vi "日志信息出发送队列 (子VI).vi"() -> (0 "错误输出":errorcluster)   [LabVIEW 2016, in "数据传输系统.lvlib"]
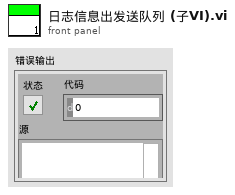
[diagram p1: front panel]
types:
  T1 = enum16{"空白测试", "跨度核查", "标样核查", "加标回收", "平行样", "集成干预"}
  T2 = cluster{"氨氮零点核查索引起始时间":string, "总磷零点核查索引起始时间":string, "总氮零点核查索引起始时间":string, "CODMn零点核查索引起始时间":string, "CODCr零点核查索引起始时间":string, "亚硝酸盐零点核查索引起始时间":string, "硫化物零点核查索引起始时间":string, "ORP零点核查索引起始时间":string}
  T3 = cluster{"数组[0]":string, "数组[1]":string, "数组[2]":string, "数组[3]":string, "数组[4]":string, "数组[5]":string, "数组[6]":string, "数组[7]":string}
  T4 = cluster{"PH":string[][], "CODCr":string[][], "氨氮":string[][], "CODMn":string[][], "总氮":string[][], "总磷":string[][], "电导率":string[][], "水温":string[][], "DO":string[][], "浊度":string[][], "叶绿素":string[][], "藻密度":string[][], "铜":string[][], "盐度":string[][], "水位":string[][], "流速":string[][], "瞬时流量":string[][], "累积流量":string[][], "亚硝酸盐":string[][], "硫化物":string[][], "ORP":string[][], "铅":string[][], "镉":string[][], "锌":string[][], "镍":string[][], "锰":string[][], "汞":string[][], "气温":string[][], "气压":string[][], "风速":string[][], "风向":string[][], "盐度 2":string[][], "磷酸盐":string[][], "硝氮":string[][]}
  T5 = cluster{"氨氮跨度核查索引起始时间":string, "总磷跨度核查索引起始时间":string, "总氮跨度核查索引起始时间":string, "CODMn跨度核查索引起始时间":string, "CODCr跨度核查索引起始时间":string, "亚硝酸盐跨度核查索引起始时间":string, "硫化物跨度核查索引起始时间":string, "ORP跨度核查索引起始时间":string}
  T6 = cluster{"氨氮标样核查索引起始时间":string, "总磷标样核查索引起始时间":string, "总氮标样核查索引起始时间":string, "CODMn标样核查索引起始时间":string, "CODCr标样核查索引起始时间":string, "DO标样核查索引起始时间":string, "PH标样核查索引起始时间":string, "比电导率标样核查索引起始时间":string, "水温标样核查索引起始时间":string, "浊度标样核查索引起始时间":string, "叶绿素a标样核查索引起始时间":string, "藻密度标样核查索引起始时间":string, "亚硝酸盐标样核查索引起始时间":string, "硫化物标样核查索引起始时间":string, "ORP标样核查索引起始时间":string}
  T7 = cluster{"数组[0]":string, "数组[1]":string, "数组[2]":string, "数组[3]":string, "数组[4]":string, "数组[5]":string, "数组[6]":string, "数组[7]":string, "数组[8]":string, "数组[9]":string, "数组[10]":string, "数组[11]":string, "数组[12]":string, "数组[13]":string, "数组[14]":string}
  T8 = cluster{"氨氮加标回收索引起始时间":string, "总磷加标回收索引起始时间":string, "总氮加标回收索引起始时间":string, "CODMn加标回收索引起始时间":string, "CODCr加标回收索引起始时间":string}
  T9 = cluster{"[0]":string, "[1]":string, "[2]":string, "[3]":string, "[4]":string}
  T10 = cluster{"氨氮平行样索引起始时间":string, "总磷平行样索引起始时间":string, "总氮平行样索引起始时间":string, "CODMn平行样索引起始时间":string, "CODCr平行样索引起始时间":string}
  T11 = cluster{"氨氮集成干预索引起始时间":string, "总磷集成干预索引起始时间":string, "总氮集成干预索引起始时间":string, "CODMn集成干预索引起始时间":string, "CODCr集成干预索引起始时间":string, "DO集成干预索引起始时间":string, "PH集成干预索引起始时间":string, "比电导率集成干预索引起始时间":string, "水温集成干预索引起始时间":string, "浊度集成干预索引起始时间":string, "叶绿素a集成干预索引起始时间":string, "藻密度集成干预索引起始时间":string, "亚硝酸盐集成干预索引起始时间":string, "硫化物集成干预索引起始时间":string, "ORP集成干预索引起始时间":string}
  T12 = cluster{"[0]":string, "[1]":string, "[2]":string, "[3]":string, "[4]":string, "[5]":string, "[6]":string, "[7]":string, "[8]":string, "[9]":string, "[10]":string, "[11]":string, "[12]":string, "[13]":string, "[14]":string}
  T13 = cluster{"氨氮仪器日志索引起始时间":string, "总磷仪器日志索引起始时间":string, "总氮仪器日志索引起始时间":string, "CODMn仪器日志索引起始时间":string, "CODCr仪器日志索引起始时间":string, "系统仪器日志索引起始时间":string}
  T14 = cluster{"[0]":string, "[1]":string, "[2]":string, "[3]":string, "[4]":string, "[5]":string}
  T15 = cluster{"氨氮报警信息索引起始时间":string, "总磷报警信息索引起始时间":string, "总氮报警信息索引起始时间":string, "CODMn报警信息索引起始时间":string, "CODCr报警信息索引起始时间":string, "DO报警信息索引起始时间":string, "PH报警信息索引起始时间":string, "比电导率报警信息索引起始时间":string, "水温报警信息索引起始时间":string, "浊度报警信息索引起始时间":string, "叶绿素报警信息索引起始时间":string, "系统报警信息索引起始时间":string}
  T16 = cluster{"[0]":string, "[1]":string, "[2]":string, "[3]":string, "[4]":string, "[5]":string, "[6]":string, "[7]":string, "[8]":string, "[9]":string, "[10]":string, "[11]":string}
  T17 = cluster{"氨氮仪器参数索引起始时间":string, "总磷仪器参数索引起始时间":string, "总氮仪器参数索引起始时间":string, "CODMn仪器参数索引起始时间":string, "CODCr仪器参数索引起始时间":string, "DO仪器参数索引起始时间":string, "PH仪器参数索引起始时间":string, "比电导率仪器参数索引起始时间":string, "水温仪器参数索引起始时间":string, "浊度仪器参数索引起始时间":string, "叶绿素a仪器参数索引起始时间":string, "藻密度仪器参数索引起始时间":string, "ORP仪器参数索引起始时间":string}
  T18 = cluster{"[0]":string, "[1]":string, "[2]":string, "[3]":string, "[4]":string, "[5]":string, "[6]":string, "[7]":string, "[8]":string, "[9]":string, "[10]":string, "[11]":string, "[12]":string}
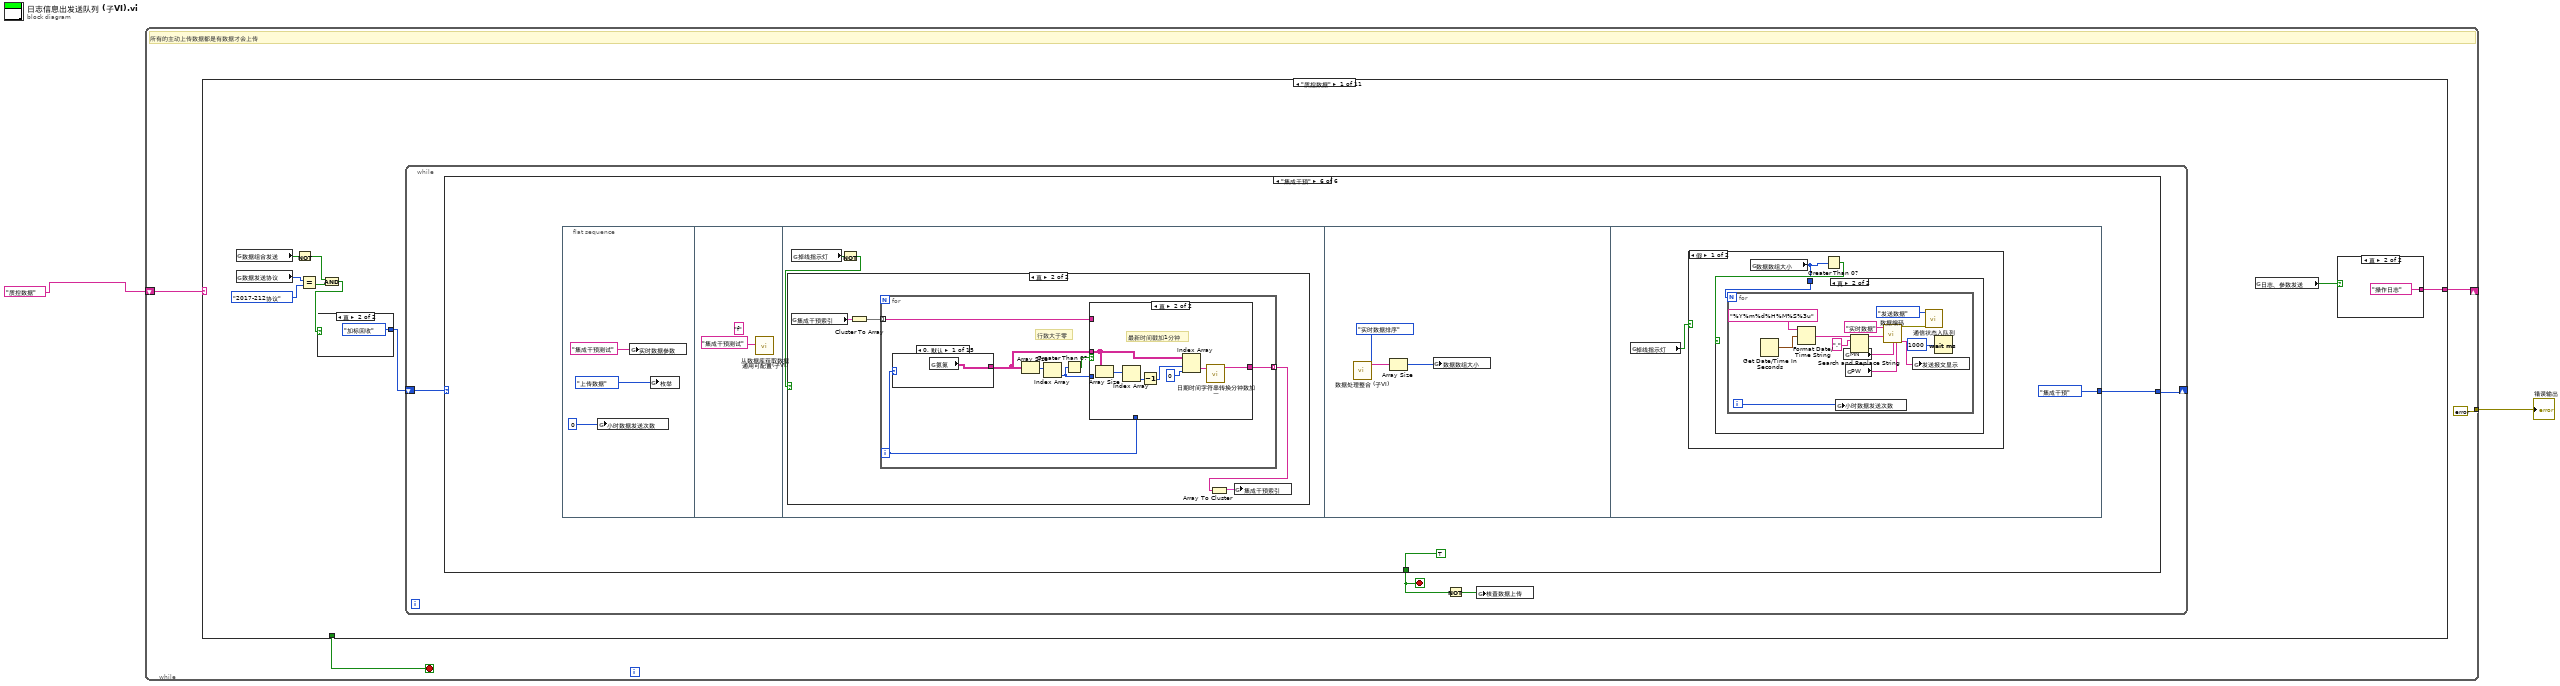
[diagram p0: block diagram]
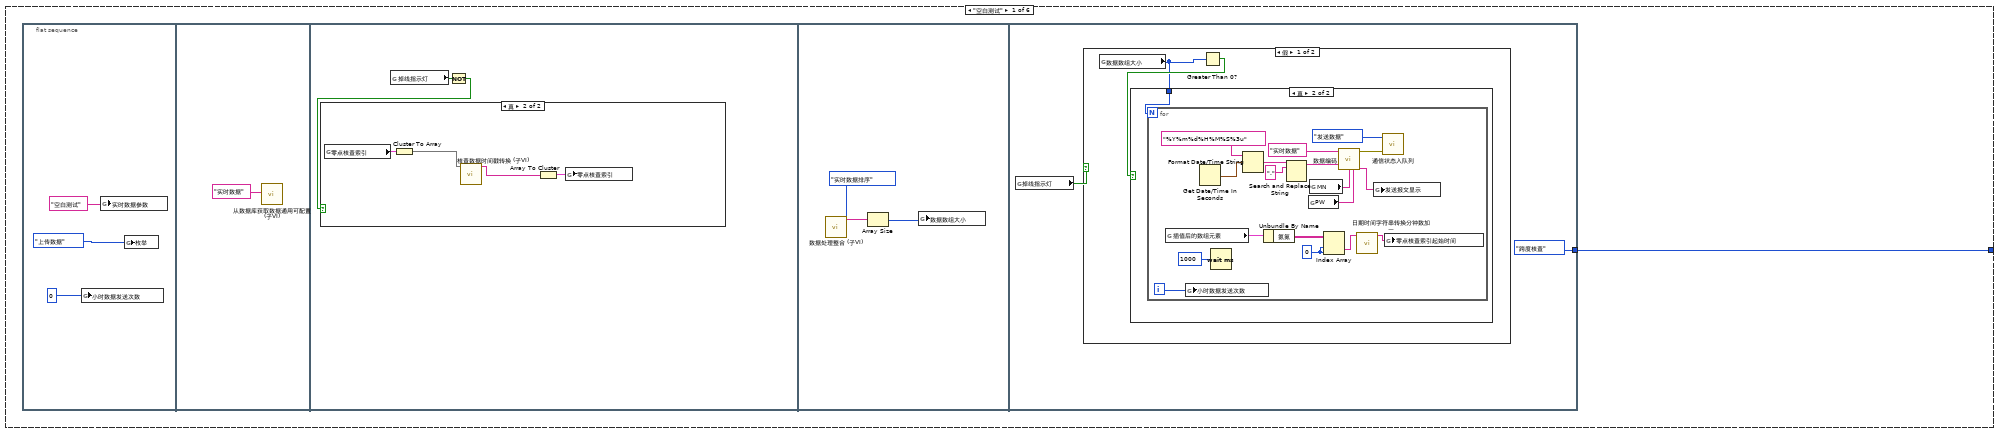
[diagram p2: hidden frame]
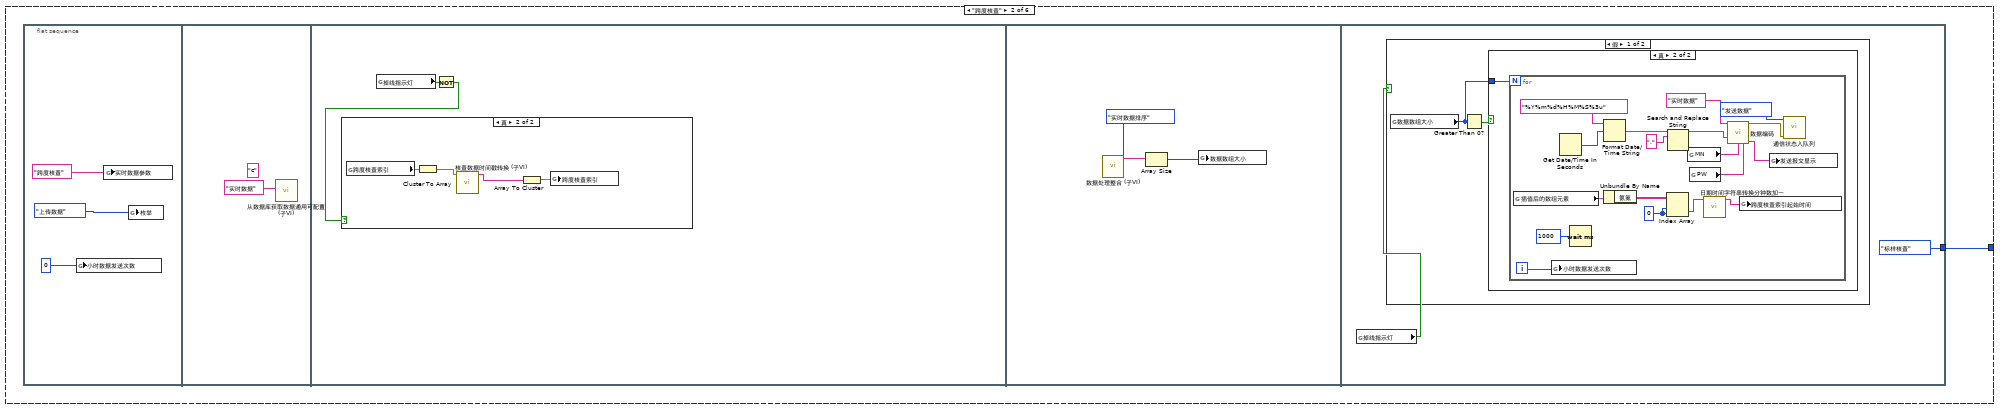
[diagram p6: hidden frame]
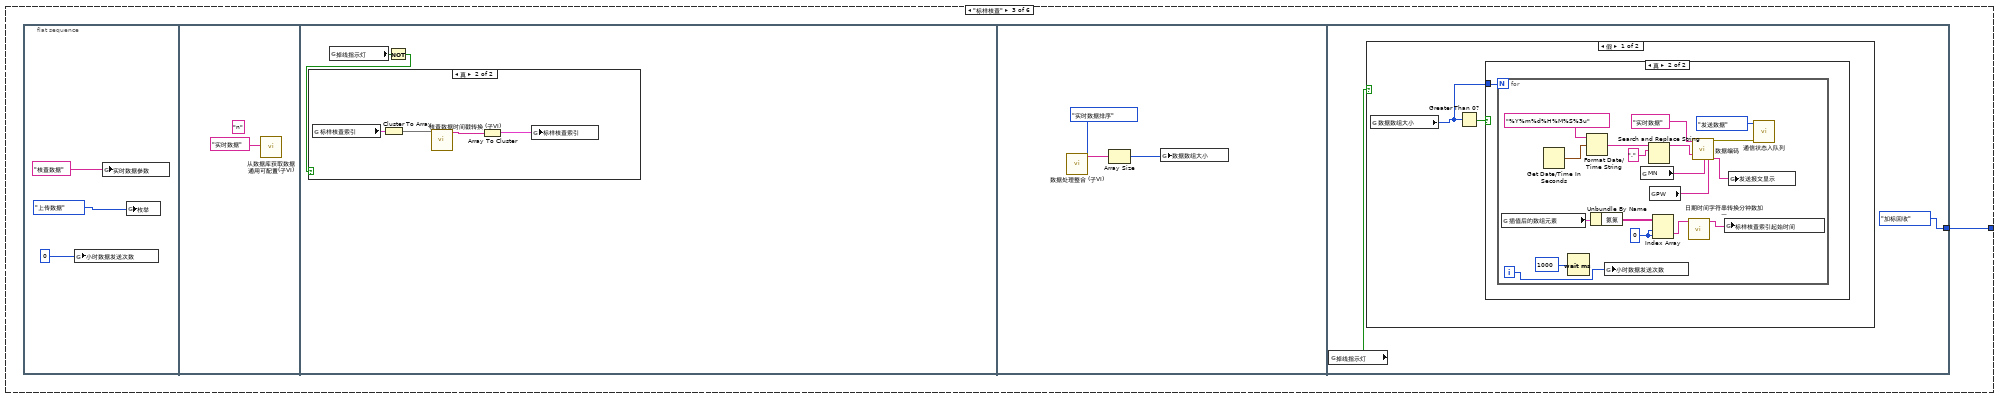
[diagram p10: hidden frame]
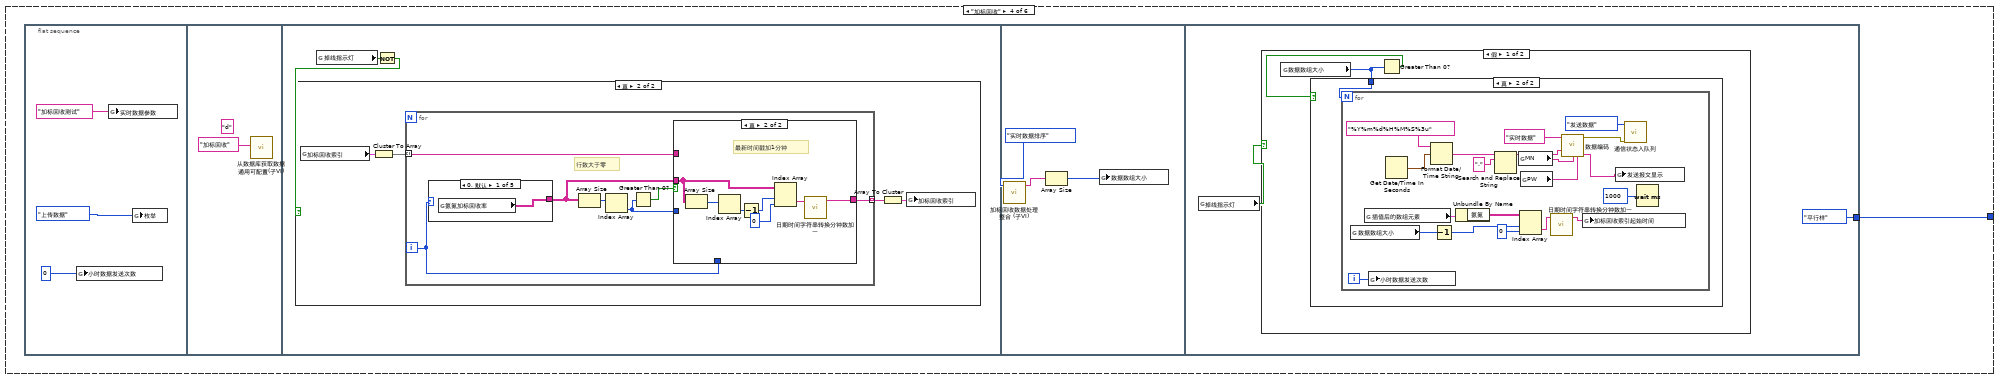
[diagram p14: hidden frame]
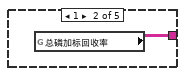
[diagram p16: hidden frame]
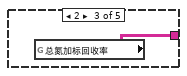
[diagram p17: hidden frame]
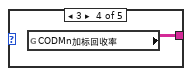
[diagram p18: hidden frame]
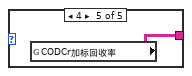
[diagram p19: hidden frame]
diagram:
  n1 = while "While循环" {
    shift-right: [w5] -> _
    shift-left: "质控数据" ("组合框") -> [w6]
    tunnel: [errorcluster {"status"=FALSE, "code"=0, "source"=""} ("错误输出")] -> w2
    stop <- w3 stop-if-true
    # "所有的主动上传数据都是有数据才会上传"
    n2 = case shown="\"质控数据\"" w6 {
      tunnel: [w15 w309 "系统状态" ("组合框") w410 "测量周期" ("组合框") "超标留样" ("组合框") "报警信息" ("组合框") w504 w569 "环境参数" ("组合框") "环境参数" ("组合框")] -> w5
      tunnel: [_ _ _ _ _ _ _ _ _ _ TRUE] -> w3
      frame "质控数据" {
        n3 = global read "断电保存全局.vi" "数据组合发送"() -> (w10:bool)
        n4 = global read "断电保存全局.vi" "数据发送协议"() -> (w13:enum16{"2005-212协议", "2017-212协议"})
        n5 = Not(x=w10) -> (.not. x?=w9:bool)
        n6 = Equal?(x=w13, y=enum16{"2005-212协议", "2017-212协议"}."2017-212协议" ("数据发送协议")) -> (x = y?=w11:bool)
        n7 = And(x=w9, y=w11) -> (x .and. y?=w8:bool)
        n8 = case shown="真" w8 {
          tunnel: [T1."空白测试" T1."加标回收"] -> w7
          frame False {
          }
          frame True {
          }
        }
        n9 = while {
          shift-right: [w18] -> _
          shift-left: w7 -> [w19]
          stop <- w16 stop-if-true
          n10 = case shown="\"集成干预\"" w19 {
            tunnel: [_ _ _ _ _ TRUE] -> w16
            tunnel: [w20 w57 w94 w131 w190 w242] -> w18
            frame "空白测试" {
              n11 = flat-sequence {
                tunnel: [T1."跨度核查"] -> w20
                frame #0 {
                  n12 = global write "全局 小时数据发送次数.vi" "小时数据发送次数"(0 ("小时数据发送次数")) -> ()
                  n13 = global write "全局 实时数据参数.vi" "实时数据参数"("空白测试") -> ()
                  n14 = global write "全局1.vi" "枚举"(enum16{"返回请求应答", "上传数据", "返回执行结果"}."上传数据" ("枚举")) -> ()
                }
                frame #1 {
                  n15 = call "从数据库获取数据通用可配置(子VI).vi"("table输入"="实时数据" ("新元素/子数组")) -> ()  [unwired: 9 in, 2 out]
                }
                frame #2 {
                  n16 = global read "全局 数据发送重叠.vi" "掉线指示灯"() -> (w26:bool)
                  n17 = Not(x=w26) -> (.not. x?=w25:bool)
                  n18 = case shown="真" w25 {
                    frame False {
                    }
                    frame True {
                      n19 = global read "全局 时间2.vi" "零点核查索引"() -> (w30:T2)
                      n20 = Cluster To Array(cluster=w30) -> (array=w28:string[])
                      n21 = call "核查数据时间戳转换 (子VI).vi"("核查索引"=w28) -> ("数组"=w27:string[])  [unwired: 10 in]
                      n22 = Array To Cluster(array=w27) -> (cluster=w29:T3)
                      n23 = global write "全局 时间2.vi" "零点核查索引"(w29) -> ()
                    }
                  }
                }
                frame #3 {
                  n24 = call "数据处理整合 (子VI).vi"("枚举"=enum16{"实时数据排序", "小时数据排序"}."实时数据排序") -> ("已排序的数组"=w33:string[])  [unwired: 10 in]
                  n25 = Array Size(array=w33) -> (size(s)=w32:i32)
                  n26 = global write "全局 数据数组大小.vi" "数据数组大小"(w32) -> ()
                }
                frame #4 {
                  n27 = global read "全局 数据发送重叠.vi" "掉线指示灯"() -> (w35:bool)
                  n28 = case shown="假" w35 {
                    frame False {
                      n29 = global read "全局 数据数组大小.vi" "数据数组大小"() -> (w36:i32)
                      n30 = Greater Than 0?(x=w36) -> (x > 0?=w37:bool)
                      n31 = case shown="真" w37 {
                        tunnel: w36 -> [_ w38]
                        frame False {
                        }
                        frame True {
                          n32 = for {
                            N: w38 -> [_]
                            i -> [w39]
                            w51 = 0 ("禁用的索引 (列)")
                            n33 = global read "插值后的新数组.vi" "插值后的数组元素"() -> (w55:T4)
                            n34 = global write "全局 小时数据发送次数.vi" "小时数据发送次数"(w39) -> ()
                            n35 = Get Date/Time In Seconds() -> (seconds since 1Jan1904=w43:timestamp)
                            n36 = Wait (ms)(milliseconds to wait=u32 1000 ("等待时间（毫秒）")) -> ()  [unwired: 1 out]
                            n37 = Format Date/Time String(time format string (%c)="%Y%m%d%H%M%S%3u" ("时间格式字符串(%c)"), seconds (now)=w43) -> (date/time string=w42:string)  [unwired: 1 in]
                            n38 = Unbundle By Name(w55) -> ("氨氮"=w54:string[][])
                            n39 = Search and Replace String(input string=w42, search string="." ("搜索字符串")) -> (result string=w40:string)  [unwired: 6 in, 3 out]
                            n40 = global read "断电保存全局.vi" "PW"() -> (w47:string)
                            n41 = global read "断电保存全局.vi" "MN"() -> (w48:string)
                            n42 = Index Array(array=w54, index (row)=w51, index (col)=w51) -> (element=w53:string)
                            n43 = call "数据编码.vi"("table输入"="实时数据" ("新元素/子数组"), "QN"=w40, "MN"=w48, "PW"=w47) -> ("错误常量"=w46:errorcluster, "通讯包字符串"=w50:string)  [unwired: 10 in]
                            n44 = call "日期时间字符串转换分钟数加一.vi"("data[0]"=w53) -> ("日期/时间字符串"=w52:string)  [unwired: 10 in]
                            n45 = global write "全局1.vi" "发送报文显示"(w50) -> ()
                            n46 = call "通信状态入队列.vi"("错误输入（无错误）"=w46, "枚举"=enum16{"打开连接", "发送数据", "读取数据", "数据处理", "关闭连接"}."发送数据") -> ()  [unwired: 9 in, 1 out]
                            n47 = global write "全局 时间2.vi" "零点核查索引起始时间"(w52) -> ()
                          }
                        }
                      }
                    }
                    frame True {
                    }
                  }
                }
              }
            }
            frame "跨度核查" {
              n48 = flat-sequence {
                tunnel: [T1."标样核查"] -> w57
                frame #0 {
                  n49 = global write "全局 小时数据发送次数.vi" "小时数据发送次数"(0 ("小时数据发送次数")) -> ()
                  n50 = global write "全局 实时数据参数.vi" "实时数据参数"("跨度核查") -> ()
                  n51 = global write "全局1.vi" "枚举"(enum16{"返回请求应答", "上传数据", "返回执行结果"}."上传数据" ("枚举")) -> ()
                }
                frame #1 {
                  (unwired) "c" ("列队名（唯一）")
                  n52 = call "从数据库获取数据通用可配置(子VI).vi"("table输入"="实时数据" ("新元素/子数组")) -> ()  [unwired: 9 in, 2 out]
                }
                frame #2 {
                  n53 = global read "全局 数据发送重叠.vi" "掉线指示灯"() -> (w63:bool)
                  n54 = Not(x=w63) -> (.not. x?=w62:bool)
                  n55 = case shown="真" w62 {
                    frame False {
                    }
                    frame True {
                      n56 = global read "全局 时间2.vi" "跨度核查索引"() -> (w67:T5)
                      n57 = Cluster To Array(cluster=w67) -> (array=w65:string[])
                      n58 = call "核查数据时间戳转换 (子VI).vi"("核查索引"=w65) -> ("数组"=w64:string[])  [unwired: 10 in]
                      n59 = Array To Cluster(array=w64) -> (cluster=w66:T3)
                      n60 = global write "全局 时间2.vi" "跨度核查索引"(w66) -> ()
                    }
                  }
                }
                frame #3 {
                  n61 = call "数据处理整合 (子VI).vi"("枚举"=enum16{"实时数据排序", "小时数据排序"}."实时数据排序") -> ("已排序的数组"=w70:string[])  [unwired: 10 in]
                  n62 = Array Size(array=w70) -> (size(s)=w69:i32)
                  n63 = global write "全局 数据数组大小.vi" "数据数组大小"(w69) -> ()
                }
                frame #4 {
                  n64 = global read "全局 数据发送重叠.vi" "掉线指示灯"() -> (w72:bool)
                  n65 = case shown="假" w72 {
                    frame False {
                      n66 = global read "全局 数据数组大小.vi" "数据数组大小"() -> (w73:i32)
                      n67 = Greater Than 0?(x=w73) -> (x > 0?=w74:bool)
                      n68 = case shown="真" w74 {
                        tunnel: w73 -> [_ w75]
                        frame False {
                        }
                        frame True {
                          n69 = for {
                            N: w75 -> [_]
                            i -> [w76]
                            w88 = 0 ("禁用的索引 (列)")
                            n70 = global read "插值后的新数组.vi" "插值后的数组元素"() -> (w92:T4)
                            n71 = global write "全局 小时数据发送次数.vi" "小时数据发送次数"(w76) -> ()
                            n72 = Get Date/Time In Seconds() -> (seconds since 1Jan1904=w80:timestamp)
                            n73 = Wait (ms)(milliseconds to wait=u32 1000 ("等待时间（毫秒）")) -> ()  [unwired: 1 out]
                            n74 = Format Date/Time String(time format string (%c)="%Y%m%d%H%M%S%3u" ("时间格式字符串(%c)"), seconds (now)=w80) -> (date/time string=w79:string)  [unwired: 1 in]
                            n75 = Unbundle By Name(w92) -> ("氨氮"=w91:string[][])
                            n76 = Index Array(array=w91, index (row)=w88, index (col)=w88) -> (element=w90:string)
                            n77 = Search and Replace String(input string=w79, search string="." ("搜索字符串")) -> (result string=w77:string)  [unwired: 6 in, 3 out]
                            n78 = global read "断电保存全局.vi" "MN"() -> (w86:string)
                            n79 = global read "断电保存全局.vi" "PW"() -> (w85:string)
                            n80 = call "日期时间字符串转换分钟数加一.vi"("data[0]"=w90) -> ("日期/时间字符串"=w89:string)  [unwired: 10 in]
                            n81 = call "数据编码.vi"("table输入"="实时数据" ("新元素/子数组"), "QN"=w77, "MN"=w86, "PW"=w85) -> ("错误常量"=w83:errorcluster, "通讯包字符串"=w84:string)  [unwired: 10 in]
                            n82 = global write "全局 时间2.vi" "跨度核查索引起始时间"(w89) -> ()
                            n83 = global write "全局1.vi" "发送报文显示"(w84) -> ()
                            n84 = call "通信状态入队列.vi"("错误输入（无错误）"=w83, "枚举"=enum16{"打开连接", "发送数据", "读取数据", "数据处理", "关闭连接"}."发送数据") -> ()  [unwired: 9 in, 1 out]
                          }
                        }
                      }
                    }
                    frame True {
                    }
                  }
                }
              }
            }
            frame "标样核查" {
              n85 = flat-sequence {
                tunnel: [T1."加标回收"] -> w94
                frame #0 {
                  n86 = global write "全局 小时数据发送次数.vi" "小时数据发送次数"(0 ("小时数据发送次数")) -> ()
                  n87 = global write "全局 实时数据参数.vi" "实时数据参数"("核查数据") -> ()
                  n88 = global write "全局1.vi" "枚举"(enum16{"返回请求应答", "上传数据", "返回执行结果"}."上传数据" ("枚举")) -> ()
                }
                frame #1 {
                  (unwired) "n" ("列队名（唯一）")
                  n89 = call "从数据库获取数据通用可配置(子VI).vi"("table输入"="实时数据" ("新元素/子数组")) -> ()  [unwired: 9 in, 2 out]
                }
                frame #2 {
                  n90 = global read "全局 数据发送重叠.vi" "掉线指示灯"() -> (w100:bool)
                  n91 = Not(x=w100) -> (.not. x?=w99:bool)
                  n92 = case shown="真" w99 {
                    frame False {
                    }
                    frame True {
                      n93 = global read "全局 时间2.vi" "标样核查索引"() -> (w104:T6)
                      n94 = Cluster To Array(cluster=w104) -> (array=w102:string[])
                      n95 = call "核查数据时间戳转换 (子VI).vi"("核查索引"=w102) -> ("数组"=w101:string[])  [unwired: 10 in]
                      n96 = Array To Cluster(array=w101) -> (cluster=w103:T7)
                      n97 = global write "全局 时间2.vi" "标样核查索引"(w103) -> ()
                    }
                  }
                }
                frame #3 {
                  n98 = call "数据处理整合 (子VI).vi"("枚举"=enum16{"实时数据排序", "小时数据排序"}."实时数据排序") -> ("已排序的数组"=w107:string[])  [unwired: 10 in]
                  n99 = Array Size(array=w107) -> (size(s)=w106:i32)
                  n100 = global write "全局 数据数组大小.vi" "数据数组大小"(w106) -> ()
                }
                frame #4 {
                  n101 = global read "全局 数据发送重叠.vi" "掉线指示灯"() -> (w109:bool)
                  n102 = case shown="假" w109 {
                    frame False {
                      n103 = global read "全局 数据数组大小.vi" "数据数组大小"() -> (w110:i32)
                      n104 = Greater Than 0?(x=w110) -> (x > 0?=w111:bool)
                      n105 = case shown="真" w111 {
                        tunnel: w110 -> [_ w112]
                        frame False {
                        }
                        frame True {
                          n106 = for {
                            N: w112 -> [_]
                            i -> [w113]
                            w125 = 0 ("禁用的索引 (列)")
                            n107 = global read "插值后的新数组.vi" "插值后的数组元素"() -> (w129:T4)
                            n108 = Get Date/Time In Seconds() -> (seconds since 1Jan1904=w117:timestamp)
                            n109 = Wait (ms)(milliseconds to wait=u32 1000 ("等待时间（毫秒）")) -> ()  [unwired: 1 out]
                            n110 = Format Date/Time String(time format string (%c)="%Y%m%d%H%M%S%3u" ("时间格式字符串(%c)"), seconds (now)=w117) -> (date/time string=w116:string)  [unwired: 1 in]
                            n111 = Unbundle By Name(w129) -> ("氨氮"=w128:string[][])
                            n112 = global write "全局 小时数据发送次数.vi" "小时数据发送次数"(w113) -> ()
                            n113 = global read "断电保存全局.vi" "MN"() -> (w122:string)
                            n114 = Search and Replace String(input string=w116, search string="." ("搜索字符串")) -> (result string=w114:string)  [unwired: 6 in, 3 out]
                            n115 = global read "断电保存全局.vi" "PW"() -> (w121:string)
                            n116 = Index Array(array=w128, index (row)=w125, index (col)=w125) -> (element=w127:string)
                            n117 = call "日期时间字符串转换分钟数加一.vi"("data[0]"=w127) -> ("日期/时间字符串"=w126:string)  [unwired: 10 in]
                            n118 = call "数据编码.vi"("table输入"="实时数据" ("新元素/子数组"), "QN"=w114, "MN"=w122, "PW"=w121) -> ("错误常量"=w120:errorcluster, "通讯包字符串"=w124:string)  [unwired: 10 in]
                            n119 = global write "全局 时间2.vi" "标样核查索引起始时间"(w126) -> ()
                            n120 = global write "全局1.vi" "发送报文显示"(w124) -> ()
                            n121 = call "通信状态入队列.vi"("错误输入（无错误）"=w120, "枚举"=enum16{"打开连接", "发送数据", "读取数据", "数据处理", "关闭连接"}."发送数据") -> ()  [unwired: 9 in, 1 out]
                          }
                        }
                      }
                    }
                    frame True {
                    }
                  }
                }
              }
            }
            frame "加标回收" {
              n122 = flat-sequence {
                tunnel: [T1."平行样"] -> w131
                frame #0 {
                  n123 = global write "全局 小时数据发送次数.vi" "小时数据发送次数"(0 ("小时数据发送次数")) -> ()
                  n124 = global write "全局 实时数据参数.vi" "实时数据参数"("加标回收测试") -> ()
                  n125 = global write "全局1.vi" "枚举"(enum16{"返回请求应答", "上传数据", "返回执行结果"}."上传数据" ("枚举")) -> ()
                }
                frame #1 {
                  (unwired) "d" ("列队名（唯一）")
                  n126 = call "从数据库获取数据通用可配置(子VI).vi"("table输入"="加标回收" ("新元素/子数组")) -> ()  [unwired: 9 in, 2 out]
                }
                frame #2 {
                  n127 = global read "全局 数据发送重叠.vi" "掉线指示灯"() -> (w137:bool)
                  n128 = Not(x=w137) -> (.not. x?=w136:bool)
                  n129 = case shown="真" w136 {
                    frame False {
                    }
                    frame True {
                      n130 = global read "全局 时间2.vi" "加标回收索引"() -> (w141:T8)
                      n131 = Cluster To Array(cluster=w141) -> (array=w140:string[])
                      n132 = for {
                        tunnel: [w143] -> w138 mode=indexing
                        tunnel: w140 -> [w142] mode=indexing
                        i -> [w144]
                        # "行数大于零"
                        n133 = case shown="0, 默认" w144 {
                          tunnel: [w149 w150 w151 w152 w153] -> w145
                          frame 0, Default {
                            n134 = global read "全局 所有参数.vi" "氨氮加标回收率"() -> (w149:string[][])
                          }
                          frame 1 {
                            n135 = global read "全局 所有参数.vi" "总磷加标回收率"() -> (w150:string[][])
                          }
                          frame 2 {
                            n136 = global read "全局 所有参数.vi" "总氮加标回收率"() -> (w151:string[][])
                          }
                          frame 3 {
                            n137 = global read "全局 所有参数.vi" "CODMn加标回收率"() -> (w152:string[][])
                          }
                          frame 4 {
                            n138 = global read "全局 所有参数.vi" "CODCr加标回收率"() -> (w153:string[][])
                          }
                        }
                        n139 = Array Size(array=w145) -> (size(s)=w147:i32[])
                        n140 = Index Array(array=w147) -> (element=w146:i32)  [unwired: 1 in]
                        n141 = Greater Than 0?(x=w146) -> (x > 0?=w148:bool)
                        n142 = case shown="真" w148 {
                          tunnel: w144 -> [_ _]
                          tunnel: w146 -> [_ _]
                          tunnel: w145 -> [_ w158]
                          tunnel: [w154 w155] -> w143
                          tunnel: w142 -> [w154 _]
                          frame False {
                          }
                          frame True {
                            # "最新时间戳加1分钟"
                            n143 = Array Size(array=w158) -> (size(s)=w160:i32[])
                            n144 = Index Array(array=w160) -> (element=w159:i32)  [unwired: 1 in]
                            n145 = Decrement(x=w159) -> (x-1=w157:i32)
                            n146 = Index Array(array=w158, index (row)=w157, index (col)=0 ("禁用的索引 (列)")) -> (element=w161:string)
                            n147 = call "日期时间字符串转换分钟数加一.vi"("data[0]"=w161) -> ("日期/时间字符串"=w155:string)  [unwired: 10 in]
                          }
                        }
                      }
                      n148 = Array To Cluster(array=w138) -> (cluster=w139:T9)
                      n149 = global write "全局 时间2.vi" "加标回收索引"(w139) -> ()
                    }
                  }
                }
                frame #3 {
                  n150 = call "加标回收数据处理整合 (子VI).vi"("枚举"=enum16{"实时数据排序", "小时数据排序"}."实时数据排序") -> ("已排序的数组"=w163:string[])  [unwired: 10 in]
                  n151 = Array Size(array=w163) -> (size(s)=w164:i32)
                  n152 = global write "全局 数据数组大小.vi" "数据数组大小"(w164) -> ()
                }
                frame #4 {
                  n153 = global read "全局 数据发送重叠.vi" "掉线指示灯"() -> (w166:bool)
                  n154 = case shown="假" w166 {
                    frame False {
                      n155 = global read "全局 数据数组大小.vi" "数据数组大小"() -> (w167:i32)
                      n156 = Greater Than 0?(x=w167) -> (x > 0?=w168:bool)
                      n157 = case shown="真" w168 {
                        tunnel: w167 -> [_ w169]
                        frame False {
                        }
                        frame True {
                          n158 = for {
                            N: w169 -> [_]
                            i -> [w170]
                            n159 = global read "全局 数据数组大小.vi" "数据数组大小"() -> (w185:i32)
                            n160 = global read "插值后的新数组.vi" "插值后的数组元素"() -> (w188:T4)
                            n161 = global write "全局 小时数据发送次数.vi" "小时数据发送次数"(w170) -> ()
                            n162 = Get Date/Time In Seconds() -> (seconds since 1Jan1904=w174:timestamp)
                            n163 = Format Date/Time String(time format string (%c)="%Y%m%d%H%M%S%3u" ("时间格式字符串(%c)"), seconds (now)=w174) -> (date/time string=w173:string)  [unwired: 1 in]
                            n164 = Decrement(x=w185) -> (x-1=w184:i32)
                            n165 = Unbundle By Name(w188) -> ("氨氮"=w187:string[][])
                            n166 = Search and Replace String(input string=w173, search string="." ("搜索字符串")) -> (result string=w171:string)  [unwired: 6 in, 3 out]
                            n167 = global read "断电保存全局.vi" "MN"() -> (w179:string)
                            n168 = Index Array(array=w187, index (row)=w184, index (col)=0 ("禁用的索引 (列)")) -> (element=w183:string)
                            n169 = global read "断电保存全局.vi" "PW"() -> (w178:string)
                            n170 = call "日期时间字符串转换分钟数加一.vi"("data[0]"=w183) -> ("日期/时间字符串"=w182:string)  [unwired: 10 in]
                            n171 = call "数据编码.vi"("table输入"="实时数据" ("新元素/子数组"), "QN"=w171, "MN"=w179, "PW"=w178) -> ("错误常量"=w177:errorcluster, "通讯包字符串"=w181:string)  [unwired: 10 in]
                            n172 = global write "全局 时间2.vi" "加标回收索引起始时间"(w182) -> ()
                            n173 = global write "全局1.vi" "发送报文显示"(w181) -> ()
                            n174 = call "通信状态入队列.vi"("错误输入（无错误）"=w177, "枚举"=enum16{"打开连接", "发送数据", "读取数据", "数据处理", "关闭连接"}."发送数据") -> ()  [unwired: 9 in, 1 out]
                            n175 = Wait (ms)(milliseconds to wait=u32 1000 ("等待时间（毫秒）")) -> ()  [unwired: 1 out]
                          }
                        }
                      }
                    }
                    frame True {
                    }
                  }
                }
              }
            }
            frame "平行样" {
              n176 = flat-sequence {
                tunnel: [T1."集成干预"] -> w190
                frame #0 {
                  n177 = global write "全局 小时数据发送次数.vi" "小时数据发送次数"(0 ("小时数据发送次数")) -> ()
                  n178 = global write "全局 实时数据参数.vi" "实时数据参数"("平行样测试") -> ()
                  n179 = global write "全局1.vi" "枚举"(enum16{"返回请求应答", "上传数据", "返回执行结果"}."上传数据" ("枚举")) -> ()
                }
                frame #1 {
                  (unwired) "e" ("列队名（唯一）")
                  n180 = call "从数据库获取数据通用可配置(子VI).vi"("table输入"="平行样测试" ("新元素/子数组")) -> ()  [unwired: 9 in, 2 out]
                }
                frame #2 {
                  n181 = global read "全局 数据发送重叠.vi" "掉线指示灯"() -> (w196:bool)
                  n182 = Not(x=w196) -> (.not. x?=w195:bool)
                  n183 = case shown="真" w195 {
                    frame False {
                    }
                    frame True {
                      n184 = global read "全局 时间2.vi" "平行样索引"() -> (w200:T10)
                      n185 = Cluster To Array(cluster=w200) -> (array=w199:string[])
                      n186 = for {
                        tunnel: [w202] -> w197 mode=indexing
                        tunnel: w199 -> [w201] mode=indexing
                        i -> [w203]
                        # "行数大于零"
                        n187 = case shown="4" w203 {
                          tunnel: [w208 w209 w210 w211 w212] -> w204
                          frame 0, Default {
                            n188 = global read "全局 所有参数.vi" "氨氮"() -> (w208:string[][])
                          }
                          frame 1 {
                            n189 = global read "全局 所有参数.vi" "总磷"() -> (w209:string[][])
                          }
                          frame 2 {
                            n190 = global read "全局 所有参数.vi" "总氮"() -> (w210:string[][])
                          }
                          frame 3 {
                            n191 = global read "全局 所有参数.vi" "CODMn"() -> (w211:string[][])
                          }
                          frame 4 {
                            n192 = global read "全局 所有参数.vi" "CODCr"() -> (w212:string[][])
                          }
                        }
                        n193 = Array Size(array=w204) -> (size(s)=w206:i32[])
                        n194 = Index Array(array=w206) -> (element=w205:i32)  [unwired: 1 in]
                        n195 = Greater Than 0?(x=w205) -> (x > 0?=w207:bool)
                        n196 = case shown="真" w207 {
                          tunnel: w203 -> [_ _]
                          tunnel: w205 -> [_ _]
                          tunnel: w204 -> [_ w217]
                          tunnel: [w213 w214] -> w202
                          tunnel: w201 -> [w213 _]
                          frame False {
                          }
                          frame True {
                            # "最新时间戳加1分钟"
                            n197 = Array Size(array=w217) -> (size(s)=w219:i32[])
                            n198 = Index Array(array=w219) -> (element=w218:i32)  [unwired: 1 in]
                            n199 = Decrement(x=w218) -> (x-1=w216:i32)
                            n200 = Index Array(array=w217, index (row)=w216, index (col)=0 ("禁用的索引 (列)")) -> (element=w220:string)
                            n201 = call "日期时间字符串转换分钟数加一.vi"("data[0]"=w220) -> ("日期/时间字符串"=w214:string)  [unwired: 10 in]
                          }
                        }
                      }
                      n202 = Array To Cluster(array=w197) -> (cluster=w198:T9)
                      n203 = global write "全局 时间2.vi" "平行样索引"(w198) -> ()
                    }
                  }
                }
                frame #3 {
                  n204 = call "数据处理整合 (子VI).vi"("枚举"=enum16{"实时数据排序", "小时数据排序"}."实时数据排序") -> ("已排序的数组"=w223:string[])  [unwired: 10 in]
                  n205 = Array Size(array=w223) -> (size(s)=w222:i32)
                  n206 = global write "全局 数据数组大小.vi" "数据数组大小"(w222) -> ()
                }
                frame #4 {
                  n207 = global read "全局 数据发送重叠.vi" "掉线指示灯"() -> (w224:bool)
                  n208 = case shown="假" w224 {
                    frame False {
                      n209 = global read "全局 数据数组大小.vi" "数据数组大小"() -> (w226:i32)
                      n210 = Greater Than 0?(x=w226) -> (x > 0?=w227:bool)
                      n211 = case shown="真" w227 {
                        tunnel: w226 -> [_ w228]
                        frame False {
                        }
                        frame True {
                          n212 = for {
                            N: w228 -> [_]
                            i -> [w229]
                            n213 = global write "全局 小时数据发送次数.vi" "小时数据发送次数"(w229) -> ()
                            n214 = Get Date/Time In Seconds() -> (seconds since 1Jan1904=w233:timestamp)
                            n215 = Format Date/Time String(time format string (%c)="%Y%m%d%H%M%S%3u" ("时间格式字符串(%c)"), seconds (now)=w233) -> (date/time string=w232:string)  [unwired: 1 in]
                            n216 = Search and Replace String(input string=w232, search string="." ("搜索字符串")) -> (result string=w230:string)  [unwired: 6 in, 3 out]
                            n217 = global read "断电保存全局.vi" "MN"() -> (w238:string)
                            n218 = global read "断电保存全局.vi" "PW"() -> (w237:string)
                            n219 = call "数据编码.vi"("table输入"="实时数据" ("新元素/子数组"), "QN"=w230, "MN"=w238, "PW"=w237) -> ("错误常量"=w236:errorcluster, "通讯包字符串"=w240:string)  [unwired: 10 in]
                            n220 = global write "全局1.vi" "发送报文显示"(w240) -> ()
                            n221 = call "通信状态入队列.vi"("错误输入（无错误）"=w236, "枚举"=enum16{"打开连接", "发送数据", "读取数据", "数据处理", "关闭连接"}."发送数据") -> ()  [unwired: 9 in, 1 out]
                            n222 = Wait (ms)(milliseconds to wait=u32 1000 ("等待时间（毫秒）")) -> ()  [unwired: 1 out]
                          }
                        }
                      }
                    }
                    frame True {
                    }
                  }
                }
              }
            }
            frame "集成干预" {
              n223 = flat-sequence {
                tunnel: [T1."集成干预"] -> w242
                frame #0 {
                  n224 = global write "全局 小时数据发送次数.vi" "小时数据发送次数"(0 ("小时数据发送次数")) -> ()
                  n225 = global write "全局 实时数据参数.vi" "实时数据参数"("集成干预测试") -> ()
                  n226 = global write "全局1.vi" "枚举"(enum16{"返回请求应答", "上传数据", "返回执行结果"}."上传数据" ("枚举")) -> ()
                }
                frame #1 {
                  (unwired) "f" ("列队名（唯一）")
                  n227 = call "从数据库获取数据通用可配置(子VI).vi"("table输入"="集成干预测试" ("新元素/子数组")) -> ()  [unwired: 9 in, 2 out]
                }
                frame #2 {
                  n228 = global read "全局 数据发送重叠.vi" "掉线指示灯"() -> (w249:bool)
                  n229 = Not(x=w249) -> (.not. x?=w248:bool)
                  n230 = case shown="真" w248 {
                    frame False {
                    }
                    frame True {
                      n231 = global read "全局 时间2.vi" "集成干预索引"() -> (w253:T11)
                      n232 = Cluster To Array(cluster=w253) -> (array=w252:string[])
                      n233 = for {
                        tunnel: [w255] -> w250 mode=indexing
                        tunnel: w252 -> [w254] mode=indexing
                        i -> [w256]
                        # "行数大于零"
                        n234 = case shown="0, 默认" w256 {
                          tunnel: [w261 w262 w263 w264 w265 w266 w267 w268 w269 w270 w271 w272 w273 w274 w275] -> w257
                          frame 0, Default {
                            n235 = global read "全局 所有参数.vi" "氨氮"() -> (w261:string[][])
                          }
                          frame 1 {
                            n236 = global read "全局 所有参数.vi" "总磷"() -> (w262:string[][])
                          }
                          frame 2 {
                            n237 = global read "全局 所有参数.vi" "总氮"() -> (w263:string[][])
                          }
                          frame 3 {
                            n238 = global read "全局 所有参数.vi" "CODMn"() -> (w264:string[][])
                          }
                          frame 4 {
                            n239 = global read "全局 所有参数.vi" "CODCr"() -> (w265:string[][])
                          }
                          frame 5 {
                            n240 = global read "全局 所有参数.vi" "DO"() -> (w266:string[][])
                          }
                          frame 6 {
                            n241 = global read "全局 所有参数.vi" "PH"() -> (w267:string[][])
                          }
                          frame 7 {
                            n242 = global read "全局 所有参数.vi" "电导率"() -> (w268:string[][])
                          }
                          frame 8 {
                            n243 = global read "全局 所有参数.vi" "水温"() -> (w269:string[][])
                          }
                          frame 9 {
                            n244 = global read "全局 所有参数.vi" "浊度"() -> (w270:string[][])
                          }
                          frame 10 {
                            n245 = global read "全局 所有参数.vi" "叶绿素"() -> (w271:string[][])
                          }
                          frame 11 {
                            n246 = global read "全局 所有参数.vi" "藻密度"() -> (w272:string[][])
                          }
                          frame 12 {
                            n247 = global read "全局 所有参数.vi" "亚硝酸盐"() -> (w273:string[][])
                          }
                          frame 13 {
                            n248 = global read "全局 所有参数.vi" "硫化物"() -> (w274:string[][])
                          }
                          frame 14 {
                            n249 = global read "全局 所有参数.vi" "ORP"() -> (w275:string[][])
                          }
                        }
                        n250 = Array Size(array=w257) -> (size(s)=w259:i32[])
                        n251 = Index Array(array=w259) -> (element=w258:i32)  [unwired: 1 in]
                        n252 = Greater Than 0?(x=w258) -> (x > 0?=w260:bool)
                        n253 = case shown="真" w260 {
                          tunnel: w256 -> [_ _]
                          tunnel: w258 -> [_ _]
                          tunnel: w257 -> [_ w278]
                          tunnel: [w276 w277] -> w255
                          tunnel: w254 -> [w276 _]
                          frame False {
                          }
                          frame True {
                            # "最新时间戳加1分钟"
                            n254 = Array Size(array=w278) -> (size(s)=w282:i32[])
                            n255 = Index Array(array=w282) -> (element=w281:i32)  [unwired: 1 in]
                            n256 = Decrement(x=w281) -> (x-1=w280:i32)
                            n257 = Index Array(array=w278, index (row)=w280, index (col)=0 ("禁用的索引 (列)")) -> (element=w283:string)
                            n258 = call "日期时间字符串转换分钟数加一.vi"("data[0]"=w283) -> ("日期/时间字符串"=w277:string)  [unwired: 10 in]
                          }
                        }
                      }
                      n259 = Array To Cluster(array=w250) -> (cluster=w251:T12)
                      n260 = global write "全局 时间2.vi" "集成干预索引"(w251) -> ()
                    }
                  }
                }
                frame #3 {
                  n261 = call "数据处理整合 (子VI).vi"("枚举"=enum16{"实时数据排序", "小时数据排序"}."实时数据排序") -> ("已排序的数组"=w286:string[])  [unwired: 10 in]
                  n262 = Array Size(array=w286) -> (size(s)=w285:i32)
                  n263 = global write "全局 数据数组大小.vi" "数据数组大小"(w285) -> ()
                }
                frame #4 {
                  n264 = global read "全局 数据发送重叠.vi" "掉线指示灯"() -> (w288:bool)
                  n265 = case shown="假" w288 {
                    frame False {
                      n266 = global read "全局 数据数组大小.vi" "数据数组大小"() -> (w289:i32)
                      n267 = Greater Than 0?(x=w289) -> (x > 0?=w290:bool)
                      n268 = case shown="真" w290 {
                        tunnel: w289 -> [_ w291]
                        frame False {
                        }
                        frame True {
                          n269 = for {
                            N: w291 -> [_]
                            i -> [w292]
                            n270 = Get Date/Time In Seconds() -> (seconds since 1Jan1904=w296:timestamp)
                            n271 = Format Date/Time String(time format string (%c)="%Y%m%d%H%M%S%3u" ("时间格式字符串(%c)"), seconds (now)=w296) -> (date/time string=w295:string)  [unwired: 1 in]
                            n272 = global write "全局 小时数据发送次数.vi" "小时数据发送次数"(w292) -> ()
                            n273 = global read "断电保存全局.vi" "MN"() -> (w300:string)
                            n274 = global read "断电保存全局.vi" "PW"() -> (w299:string)
                            n275 = Search and Replace String(input string=w295, search string="." ("搜索字符串")) -> (result string=w293:string)  [unwired: 6 in, 3 out]
                            n276 = call "数据编码.vi"("table输入"="实时数据" ("新元素/子数组"), "QN"=w293, "MN"=w300, "PW"=w299) -> ("错误常量"=w301:errorcluster, "通讯包字符串"=w303:string)  [unwired: 10 in]
                            n277 = global write "全局1.vi" "发送报文显示"(w303) -> ()
                            n278 = call "通信状态入队列.vi"("错误输入（无错误）"=w301, "枚举"=enum16{"打开连接", "发送数据", "读取数据", "数据处理", "关闭连接"}."发送数据") -> ()  [unwired: 9 in, 1 out]
                            n279 = Wait (ms)(milliseconds to wait=u32 1000 ("等待时间（毫秒）")) -> ()  [unwired: 1 out]
                          }
                        }
                      }
                    }
                    frame True {
                    }
                  }
                }
              }
            }
          }
          n280 = Not(x=w16) -> (.not. x?=w17:bool)
          n281 = global write "全局1.vi" "核查数据上传"(w17) -> ()
        }
        n282 = global read "断电保存全局.vi" "日志、参数发送"() -> (w14:bool)
        n283 = case shown="真" w14 {
          tunnel: ["环境参数" ("组合框") "操作日志" ("组合框")] -> w15
          frame False {
          }
          frame True {
          }
        }
      }
      frame "操作日志" {
        # "间隔时间上传"
        # "直接1分钟查询 一次,有数据就按数据上传,没数据就不上传,在数据发送那边有做处理"
        n284 = flat-sequence {
          frame #0 {
            # "时间"
            n285 = global write "全局 小时数据发送次数.vi" "小时数据发送次数"(0 ("小时数据发送次数")) -> ()
            n286 = call "日志信息主动发送(子VI).vi"() -> ()  [unwired: 12 in]
            n287 = global write "全局1.vi" "枚举"(enum16{"返回请求应答", "上传数据", "返回执行结果"}."上传数据" ("枚举")) -> ()
          }
          frame #1 {
            n288 = call "获取操作日志 (子VI).vi"("table输入"="操作日志") -> ()  [unwired: 11 in]
          }
          frame #2 {
            n289 = call "数据处理整合 (子VI).vi"("枚举"=enum16{"实时数据排序", "小时数据排序"}."实时数据排序") -> ("已排序的数组"=w318:string[])  [unwired: 10 in]
            n290 = Array Size(array=w318) -> (size(s)=w317:i32)
            n291 = global write "全局 数据数组大小.vi" "数据数组大小"(w317) -> ()
          }
          frame #3 {
            n292 = global read "全局 数据发送重叠.vi" "掉线指示灯"() -> (w320:bool)
            n293 = Not(x=w320) -> (.not. x?=w319:bool)
            n294 = case shown="真" w319 {
              frame False {
              }
              frame True {
                n295 = global read "全局 时间2.vi" "仪器日志索引"() -> (w324:T13)
                n296 = Cluster To Array(cluster=w324) -> (array=w323:string[])
                n297 = for {
                  tunnel: w323 -> [w325] mode=indexing
                  tunnel: [w326] -> w321 mode=indexing
                  i -> [w328]
                  # "行数大于零"
                  n298 = case shown="5" w328 {
                    tunnel: [w332 w333 w334 w335 w336 w337] -> w327
                    frame 0, Default {
                      n299 = global read "全局 所有参数.vi" "氨氮"() -> (w332:string[][])
                    }
                    frame 1 {
                      n300 = global read "全局 所有参数.vi" "总磷"() -> (w333:string[][])
                    }
                    frame 2 {
                      n301 = global read "全局 所有参数.vi" "总氮"() -> (w334:string[][])
                    }
                    frame 3 {
                      n302 = global read "全局 所有参数.vi" "CODMn"() -> (w335:string[][])
                    }
                    frame 4 {
                      n303 = global read "全局 所有参数.vi" "CODCr"() -> (w336:string[][])
                    }
                    frame 5 {
                      n304 = global read "全局 所有参数.vi" "DO"() -> (w337:string[][])
                    }
                  }
                  n305 = Array Size(array=w327) -> (size(s)=w330:i32[])
                  n306 = Index Array(array=w330) -> (element=w329:i32)  [unwired: 1 in]
                  n307 = Greater Than 0?(x=w329) -> (x > 0?=w331:bool)
                  n308 = case shown="真" w331 {
                    tunnel: w329 -> [_ _]
                    tunnel: w327 -> [_ w343]
                    tunnel: [w338 w339] -> w326
                    tunnel: w325 -> [w338 _]
                    frame False {
                    }
                    frame True {
                      # "最新时间戳加1分钟"
                      n309 = Array Size(array=w343) -> (size(s)=w345:i32[])
                      n310 = Index Array(array=w345) -> (element=w344:i32)  [unwired: 1 in]
                      n311 = Decrement(x=w344) -> (x-1=w342:i32)
                      n312 = Index Array(array=w343, index (row)=w342, index (col)=0 ("禁用的索引 (列)")) -> (element=w340:string)
                      n313 = call "日期时间字符串转换秒数加一.vi"("data[0]"=w340) -> ("日期/时间字符串"=w339:string)  [unwired: 10 in]
                    }
                  }
                }
                n314 = Array To Cluster(array=w321) -> (cluster=w322:T14)
                n315 = global write "全局 时间2.vi" "仪器日志索引"(w322) -> ()
              }
            }
          }
          frame #4 {
            # "判定是否存表"
            n316 = global read "全局 数据发送重叠.vi" "掉线指示灯"() -> (w346:bool)
            n317 = case shown="假" w346 {
              frame False {
                n318 = global read "全局 数据数组大小.vi" "数据数组大小"() -> (w347:i32)
                n319 = Greater Than 0?(x=w347) -> (x > 0?=w348:bool)
                n320 = case shown="真" w348 {
                  frame False {
                  }
                  frame True {
                    n321 = while {
                      stop <- w350 stop-if-true
                      n322 = Get Date/Time In Seconds() -> (seconds since 1Jan1904=w362:timestamp)
                      n323 = Format Date/Time String(time format string (%c)="%Y%m%d%H%M%S%3u" ("时间格式字符串(%c)"), seconds (now)=w362) -> (date/time string=w361:string)  [unwired: 1 in]
                      n324 = Search and Replace String(input string=w361, search string="." ("搜索字符串")) -> (result string=w359:string)  [unwired: 6 in, 3 out]
                      n325 = global read "断电保存全局.vi" "MN"() -> (w356:string)
                      n326 = global read "断电保存全局.vi" "PW"() -> (w355:string)
                      n327 = call "数据编码.vi"("table输入"="操作日志" ("新元素/子数组"), "QN"=w359, "MN"=w356, "PW"=w355) -> ("错误常量"=w354:errorcluster, "通讯包字符串"=w358:string)  [unwired: 10 in]
                      n328 = global read "全局 小时数据发送次数.vi" "小时数据发送次数"() -> (w351:i32)
                      n329 = global read "全局 数据数组大小.vi" "数据数组大小"() -> (w352:i32)
                      n330 = call "通信状态入队列.vi"("错误输入（无错误）"=w354, "枚举"=enum16{"打开连接", "发送数据", "读取数据", "数据处理", "关闭连接"}."发送数据") -> ()  [unwired: 9 in, 1 out]
                      n331 = global write "全局1.vi" "发送报文显示"(w358) -> ()
                      n332 = Decrement(x=w352) -> (x-1=w353:i32)
                      n333 = Greater Or Equal?(x=w351, y=w353) -> (x >= y?=w350:bool)
                      n334 = Wait (ms)(milliseconds to wait=u32 1000 ("等待时间（毫秒）")) -> ()  [unwired: 1 out]
                    }
                  }
                }
              }
              frame True {
              }
            }
          }
        }
        n335 = global read "断电保存全局.vi" "应用环境"() -> (w310:enum16{"STD", "GB212"})
        n336 = case shown="\"STD\", 默认" w310 {
          tunnel: ["3092日志信息" ("组合框") "系统状态" ("组合框")] -> w309
          frame "STD", Default {
          }
          frame "GB212" {
          }
        }
      }
      frame "3092日志信息" {
        # "间隔时间上传"
        # "直接1分钟查询 一次,有数据就按数据上传,没数据就不上传,在数据发送那边有做处理"
        n337 = flat-sequence {
          tunnel: [w369] -> w365
          tunnel: w365 -> [w373]
          frame #0 {
            n338 = global write "全局 小时数据发送次数.vi" "小时数据发送次数"(0 ("小时数据发送次数")) -> ()
            n339 = global write "全局1.vi" "枚举"(enum16{"返回请求应答", "上传数据", "返回执行结果"}."上传数据" ("枚举")) -> ()
          }
          frame #1 {
            n340 = call "数据表比对.vi"("table输入"="3092日志信息") -> ("待发送数据"=w369:string[][])  [unwired: 7 in, 3 out]
            n341 = global write "全局 所有参数.vi" "CODMn"(w369) -> ()
          }
          frame #2 {
            n342 = Array Size(array=w373) -> (size(s)=w372:i32[])
            n343 = Index Array(array=w372) -> (element=w371:i32)  [unwired: 1 in]
            n344 = global write "全局 数据数组大小.vi" "数据数组大小"(w371) -> ()
          }
          frame #3 {
            n345 = global read "全局 数据发送重叠.vi" "掉线指示灯"() -> (w375:bool)
            n346 = Not(x=w375) -> (.not. x?=w374:bool)
            n347 = case shown="真" w374 {
              frame False {
              }
              frame True {
                # "行数大于零"
                n348 = global read "全局 时间2.vi" "3092日志索引起始时间"() -> (w377:string)
                n349 = global read "全局 所有参数.vi" "CODMn"() -> (w378:string[][])
                n350 = Array Size(array=w378) -> (size(s)=w380:i32[])
                n351 = Index Array(array=w380) -> (element=w379:i32)  [unwired: 1 in]
                n352 = Greater Than 0?(x=w379) -> (x > 0?=w381:bool)
                n353 = case shown="真" w381 {
                  tunnel: w379 -> [_ _]
                  tunnel: w378 -> [_ w387]
                  tunnel: [w382 w383] -> w376
                  tunnel: w377 -> [w382 _]
                  frame False {
                  }
                  frame True {
                    # "最新时间戳加1分钟"
                    n354 = Array Size(array=w387) -> (size(s)=w389:i32[])
                    n355 = Index Array(array=w389) -> (element=w388:i32)  [unwired: 1 in]
                    n356 = Decrement(x=w388) -> (x-1=w386:i32)
                    n357 = Index Array(array=w387, index (row)=w386, index (col)=0 ("禁用的索引 (列)")) -> (element=w384:string)
                    n358 = call "日期时间字符串转换秒数加一.vi"("data[0]"=w384) -> ("日期/时间字符串"=w383:string)  [unwired: 10 in]
                  }
                }
                n359 = global write "全局 时间2.vi" "3092日志索引起始时间"(w376) -> ()
              }
            }
          }
          frame #4 {
            # "判定是否存表"
            n360 = global read "全局 数据发送重叠.vi" "掉线指示灯"() -> (w390:bool)
            n361 = case shown="假" w390 {
              frame False {
                n362 = global read "全局 数据数组大小.vi" "数据数组大小"() -> (w391:i32)
                n363 = Greater Than 0?(x=w391) -> (x > 0?=w392:bool)
                n364 = case shown="真" w392 {
                  frame False {
                  }
                  frame True {
                    n365 = while {
                      stop <- w394 stop-if-true
                      n366 = global read "全局 数据数组大小.vi" "数据数组大小"() -> (w396:i32)
                      n367 = Wait (ms)(milliseconds to wait=u32 1000 ("等待时间（毫秒）")) -> ()  [unwired: 1 out]
                      n368 = global read "全局 小时数据发送次数.vi" "小时数据发送次数"() -> (w395:i32)
                      n369 = Decrement(x=w396) -> (x-1=w397:i32)
                      n370 = Greater Or Equal?(x=w395, y=w397) -> (x >= y?=w394:bool)
                      n371 = Get Date/Time In Seconds() -> (seconds since 1Jan1904=w406:timestamp)
                      n372 = Format Date/Time String(time format string (%c)="%Y%m%d%H%M%S%3u" ("时间格式字符串(%c)"), seconds (now)=w406) -> (date/time string=w405:string)  [unwired: 1 in]
                      n373 = Search and Replace String(input string=w405, search string="." ("搜索字符串")) -> (result string=w403:string)  [unwired: 6 in, 3 out]
                      n374 = global read "断电保存全局.vi" "MN"() -> (w400:string)
                      n375 = global read "断电保存全局.vi" "PW"() -> (w399:string)
                      n376 = call "数据编码.vi"("table输入"="3092日志信息" ("新元素/子数组"), "QN"=w403, "MN"=w400, "PW"=w399) -> ("错误常量"=w398:errorcluster, "通讯包字符串"=w402:string)  [unwired: 10 in]
                      n377 = call "通信状态入队列.vi"("错误输入（无错误）"=w398, "枚举"=enum16{"打开连接", "发送数据", "读取数据", "数据处理", "关闭连接"}."发送数据") -> ()  [unwired: 9 in, 1 out]
                      n378 = global write "全局1.vi" "发送报文显示"(w402) -> ()
                    }
                  }
                }
              }
              frame True {
              }
            }
          }
        }
      }
      frame "系统状态" {
        # "直接1分钟查询 一次,有变化就按上传,没变化就不上传"
        n379 = flat-sequence {
          frame #0 {
            # "时间"
            n380 = global write "全局 小时数据发送次数.vi" "小时数据发送次数"(0 ("小时数据发送次数")) -> ()
            n381 = global write "全局 数据数组大小.vi" "数据数组大小"(1 ("数据数组大小")) -> ()
            n382 = global write "全局1.vi" "枚举"(enum16{"返回请求应答", "上传数据", "返回执行结果"}."上传数据" ("枚举")) -> ()
          }
          frame #1 {
            # "判定是否存表"
            n383 = global read "全局 数据发送重叠.vi" "掉线指示灯"() -> (w416:bool)
            n384 = case shown="假" w416 {
              frame False {
                n385 = global read "全局1.vi" "系统状态"() -> (w417:bool)
                n386 = case shown="真" w417 {
                  frame False {
                  }
                  frame True {
                    n387 = for {
                      N: 6 -> [_]
                      n388 = flat-sequence {
                        frame #0 {
                          n389 = Get Date/Time In Seconds() -> (seconds since 1Jan1904=w429:timestamp)
                          n390 = Format Date/Time String(time format string (%c)="%Y%m%d%H%M%S%3u" ("时间格式字符串(%c)"), seconds (now)=w429) -> (date/time string=w428:string)  [unwired: 1 in]
                          n391 = Search and Replace String(input string=w428, search string="." ("搜索字符串")) -> (result string=w426:string)  [unwired: 6 in, 3 out]
                          n392 = global read "断电保存全局.vi" "MN"() -> (w423:string)
                          n393 = global read "断电保存全局.vi" "PW"() -> (w422:string)
                          n394 = call "数据编码.vi"("table输入"="系统状态" ("新元素/子数组"), "QN"=w426, "MN"=w423, "PW"=w422) -> ("错误常量"=w421:errorcluster, "通讯包字符串"=w425:string)  [unwired: 10 in]
                          n395 = global write "全局1.vi" "发送报文显示"(w425) -> ()
                          n396 = call "通信状态入队列.vi"("错误输入（无错误）"=w421, "枚举"=enum16{"打开连接", "发送数据", "读取数据", "数据处理", "关闭连接"}."发送数据") -> ()  [unwired: 9 in, 1 out]
                        }
                        frame #1 {
                          n397 = global read "全局 小时数据发送次数.vi" "小时数据发送次数"() -> (w433:i32)
                          n398 = Increment(x=w433) -> (x+1=w432:i32)
                          n399 = global write "全局 小时数据发送次数.vi" "小时数据发送次数"(w432) -> ()
                        }
                      }
                      n400 = Wait (ms)(milliseconds to wait=u32 1000 ("等待时间（毫秒）")) -> ()  [unwired: 1 out]
                    }
                    n401 = global write "全局1.vi" "系统状态"(FALSE ("系统状态")) -> ()
                  }
                }
              }
              frame True {
              }
            }
          }
        }
        n402 = global read "断电保存全局.vi" "应用环境"() -> (w409:enum16{"STD", "GB212"})
        n403 = case shown="\"GB212\"" w409 {
          tunnel: ["运行模式" ("组合框") "超标留样" ("组合框")] -> w410
          frame "STD", Default {
          }
          frame "GB212" {
          }
        }
      }
      frame "运行模式" {
        # "直接1分钟查询 一次,有变化就按上传,没变化就不上传"
        n404 = flat-sequence {
          frame #0 {
            # "时间"
            n405 = global write "全局 小时数据发送次数.vi" "小时数据发送次数"(0 ("小时数据发送次数")) -> ()
            n406 = global write "全局 数据数组大小.vi" "数据数组大小"(1 ("数据数组大小")) -> ()
            n407 = global write "全局1.vi" "枚举"(enum16{"返回请求应答", "上传数据", "返回执行结果"}."上传数据" ("枚举")) -> ()
          }
          frame #1 {
            # "判定是否存表"
            n408 = global read "全局 数据发送重叠.vi" "掉线指示灯"() -> (w438:bool)
            n409 = case shown="假" w438 {
              frame False {
                n410 = global read "全局1.vi" "运行模式"() -> (w439:bool)
                n411 = case shown="真" w439 {
                  frame False {
                  }
                  frame True {
                    n412 = global read "全局 小时数据发送次数.vi" "小时数据发送次数"() -> (w447:i32)
                    n413 = global write "全局1.vi" "运行模式"(FALSE ("系统状态")) -> ()
                    n414 = Get Date/Time In Seconds() -> (seconds since 1Jan1904=w451:timestamp)
                    n415 = Increment(x=w447) -> (x+1=w446:i32)
                    n416 = Format Date/Time String(time format string (%c)="%Y%m%d%H%M%S%3u" ("时间格式字符串(%c)"), seconds (now)=w451) -> (date/time string=w450:string)  [unwired: 1 in]
                    n417 = global write "全局 小时数据发送次数.vi" "小时数据发送次数"(w446) -> ()
                    n418 = Search and Replace String(input string=w450, search string="." ("搜索字符串")) -> (result string=w448:string)  [unwired: 6 in, 3 out]
                    n419 = global read "断电保存全局.vi" "MN"() -> (w443:string)
                    n420 = global read "断电保存全局.vi" "PW"() -> (w442:string)
                    n421 = call "数据编码.vi"("table输入"="运行模式" ("新元素/子数组"), "QN"=w448, "MN"=w443, "PW"=w442) -> ("错误常量"=w441:errorcluster, "通讯包字符串"=w445:string)  [unwired: 10 in]
                    n422 = call "通信状态入队列.vi"("错误输入（无错误）"=w441, "枚举"=enum16{"打开连接", "发送数据", "读取数据", "数据处理", "关闭连接"}."发送数据") -> ()  [unwired: 9 in, 1 out]
                    n423 = global write "全局1.vi" "发送报文显示"(w445) -> ()
                  }
                }
              }
              frame True {
              }
            }
          }
        }
      }
      frame "测量周期" {
        # "直接1分钟查询 一次,有变化就按上传,没变化就不上传"
        n424 = flat-sequence {
          frame #0 {
            # "时间"
            n425 = global write "全局 小时数据发送次数.vi" "小时数据发送次数"(0 ("小时数据发送次数")) -> ()
            n426 = global write "全局 数据数组大小.vi" "数据数组大小"(1 ("数据数组大小")) -> ()
            n427 = global write "全局1.vi" "枚举"(enum16{"返回请求应答", "上传数据", "返回执行结果"}."上传数据" ("枚举")) -> ()
          }
          frame #1 {
            # "判定是否存表"
            n428 = global read "全局 数据发送重叠.vi" "掉线指示灯"() -> (w458:bool)
            n429 = case shown="假" w458 {
              frame False {
                n430 = global read "全局1.vi" "测量周期"() -> (w459:bool)
                n431 = case shown="真" w459 {
                  frame False {
                  }
                  frame True {
                    n432 = flat-sequence {
                      frame #0 {
                        n433 = Get Date/Time In Seconds() -> (seconds since 1Jan1904=w469:timestamp)
                        n434 = Format Date/Time String(time format string (%c)="%Y%m%d%H%M%S%3u" ("时间格式字符串(%c)"), seconds (now)=w469) -> (date/time string=w468:string)  [unwired: 1 in]
                        n435 = global read "断电保存全局.vi" "MN"() -> (w463:string)
                        n436 = global read "断电保存全局.vi" "PW"() -> (w462:string)
                        n437 = Search and Replace String(input string=w468, search string="." ("搜索字符串")) -> (result string=w466:string)  [unwired: 6 in, 3 out]
                        n438 = call "数据编码.vi"("table输入"="测量周期" ("新元素/子数组"), "QN"=w466, "MN"=w463, "PW"=w462) -> ("错误常量"=w461:errorcluster, "通讯包字符串"=w465:string)  [unwired: 10 in]
                        n439 = call "通信状态入队列.vi"("错误输入（无错误）"=w461, "枚举"=enum16{"打开连接", "发送数据", "读取数据", "数据处理", "关闭连接"}."发送数据") -> ()  [unwired: 9 in, 1 out]
                        n440 = global write "全局1.vi" "发送报文显示"(w465) -> ()
                      }
                      frame #1 {
                        n441 = Wait (ms)(milliseconds to wait=u32 1000 ("等待时间（毫秒）")) -> ()  [unwired: 1 out]
                      }
                      frame #2 {
                        n442 = Get Date/Time In Seconds() -> (seconds since 1Jan1904=w475:timestamp)
                        n443 = Format Date/Time String(time format string (%c)="%Y%m%d%H%M%S%3u" ("时间格式字符串(%c)"), seconds (now)=w475) -> (date/time string=w476:string)  [unwired: 1 in]
                        n444 = global read "断电保存全局.vi" "MN"() -> (w481:string)
                        n445 = global read "断电保存全局.vi" "PW"() -> (w482:string)
                        n446 = Search and Replace String(input string=w476, search string="." ("搜索字符串")) -> (result string=w478:string)  [unwired: 6 in, 3 out]
                        n447 = call "数据编码.vi"("table输入"="各参数测量周期" ("新元素/子数组"), "QN"=w478, "MN"=w481, "PW"=w482) -> ("错误常量"=w483:errorcluster, "通讯包字符串"=w479:string)  [unwired: 10 in]
                        n448 = call "通信状态入队列.vi"("错误输入（无错误）"=w483, "枚举"=enum16{"打开连接", "发送数据", "读取数据", "数据处理", "关闭连接"}."发送数据") -> ()  [unwired: 9 in, 1 out]
                        n449 = global write "全局1.vi" "发送报文显示"(w479) -> ()
                      }
                    }
                    n450 = global write "全局1.vi" "测量周期"(FALSE ("系统状态")) -> ()
                  }
                }
              }
              frame True {
              }
            }
          }
        }
      }
      frame "超标留样" {
        # "直接1分钟查询 一次,有变化就按上传,没变化就不上传"
        n451 = flat-sequence {
          frame #0 {
            # "时间"
            n452 = global write "全局 小时数据发送次数.vi" "小时数据发送次数"(0 ("小时数据发送次数")) -> ()
            n453 = global write "全局 数据数组大小.vi" "数据数组大小"(1 ("数据数组大小")) -> ()
            n454 = global write "全局1.vi" "枚举"(enum16{"返回请求应答", "上传数据", "返回执行结果"}."上传数据" ("枚举")) -> ()
          }
          frame #1 {
            # "判定是否存表"
            n455 = global read "全局 数据发送重叠.vi" "掉线指示灯"() -> (w488:bool)
            n456 = case shown="假" w488 {
              frame False {
                n457 = global read "全局1.vi" "超标留样"() -> (w489:bool)
                n458 = case shown="真" w489 {
                  frame False {
                  }
                  frame True {
                    n459 = global read "全局 小时数据发送次数.vi" "小时数据发送次数"() -> (w497:i32)
                    n460 = global write "全局1.vi" "超标留样"(FALSE ("系统状态")) -> ()
                    n461 = Get Date/Time In Seconds() -> (seconds since 1Jan1904=w501:timestamp)
                    n462 = Increment(x=w497) -> (x+1=w496:i32)
                    n463 = Format Date/Time String(time format string (%c)="%Y%m%d%H%M%S%3u" ("时间格式字符串(%c)"), seconds (now)=w501) -> (date/time string=w500:string)  [unwired: 1 in]
                    n464 = global write "全局 小时数据发送次数.vi" "小时数据发送次数"(w496) -> ()
                    n465 = Search and Replace String(input string=w500, search string="." ("搜索字符串")) -> (result string=w498:string)  [unwired: 6 in, 3 out]
                    n466 = global read "断电保存全局.vi" "MN"() -> (w492:string)
                    n467 = global read "断电保存全局.vi" "PW"() -> (w491:string)
                    n468 = call "数据编码.vi"("table输入"="超标留样" ("新元素/子数组"), "QN"=w498, "MN"=w492, "PW"=w491) -> ("错误常量"=w493:errorcluster, "通讯包字符串"=w495:string)  [unwired: 10 in]
                    n469 = global write "全局1.vi" "发送报文显示"(w495) -> ()
                    n470 = call "通信状态入队列.vi"("错误输入（无错误）"=w493, "枚举"=enum16{"打开连接", "发送数据", "读取数据", "数据处理", "关闭连接"}."发送数据") -> ()  [unwired: 9 in, 1 out]
                  }
                }
              }
              frame True {
              }
            }
          }
        }
      }
      frame "报警信息" {
        # "间隔时间上传"
        # "直接1分钟查询 一次,有数据就按数据上传,没数据为空的不传,在数据发送那边有做处理"
        n471 = flat-sequence {
          frame #0 {
            # "分钟时间间隔"
            n472 = call "日志信息主动发送(子VI).vi"() -> ()  [unwired: 12 in]
            n473 = global write "全局 小时数据发送次数.vi" "小时数据发送次数"(0 ("小时数据发送次数")) -> ()
            n474 = global write "全局1.vi" "枚举"(enum16{"返回请求应答", "上传数据", "返回执行结果"}."上传数据" ("枚举")) -> ()
          }
          frame #1 {
            n475 = call "获取报警信息 (子VI).vi"() -> ()  [unwired: 12 in]
          }
          frame #2 {
            n476 = call "数据处理整合 (子VI).vi"("枚举"=enum16{"实时数据排序", "小时数据排序"}."实时数据排序") -> ("已排序的数组"=w515:string[])  [unwired: 10 in]
            n477 = Array Size(array=w515) -> (size(s)=w514:i32)
            n478 = global write "全局 数据数组大小.vi" "数据数组大小"(w514) -> ()
          }
          frame #3 {
            n479 = global read "全局 数据发送重叠.vi" "掉线指示灯"() -> (w517:bool)
            n480 = Not(x=w517) -> (.not. x?=w516:bool)
            n481 = case shown="真" w516 {
              frame False {
              }
              frame True {
                n482 = global read "全局 时间2.vi" "报警信息索引"() -> (w521:T15)
                n483 = Cluster To Array(cluster=w521) -> (array=w520:string[])
                n484 = for {
                  tunnel: [w523] -> w518 mode=indexing
                  tunnel: w520 -> [w522] mode=indexing
                  i -> [w525]
                  # "行数大于零"
                  n485 = case shown="5" w525 {
                    tunnel: [w529 w530 w531 w532 w533 w534 w535 w536 w537 w538 w539 w540] -> w524
                    frame 0, Default {
                      n486 = global read "全局 所有参数.vi" "氨氮"() -> (w529:string[][])
                    }
                    frame 1 {
                      n487 = global read "全局 所有参数.vi" "总磷"() -> (w530:string[][])
                    }
                    frame 2 {
                      n488 = global read "全局 所有参数.vi" "总氮"() -> (w531:string[][])
                    }
                    frame 3 {
                      n489 = global read "全局 所有参数.vi" "CODMn"() -> (w532:string[][])
                    }
                    frame 4 {
                      n490 = global read "全局 所有参数.vi" "CODCr"() -> (w533:string[][])
                    }
                    frame 5 {
                      n491 = global read "全局 所有参数.vi" "DO"() -> (w534:string[][])
                    }
                    frame 6 {
                      n492 = global read "全局 所有参数.vi" "PH"() -> (w535:string[][])
                    }
                    frame 7 {
                      n493 = global read "全局 所有参数.vi" "电导率"() -> (w536:string[][])
                    }
                    frame 8 {
                      n494 = global read "全局 所有参数.vi" "水温"() -> (w537:string[][])
                    }
                    frame 9 {
                      n495 = global read "全局 所有参数.vi" "浊度"() -> (w538:string[][])
                    }
                    frame 10 {
                      n496 = global read "全局 所有参数.vi" "叶绿素"() -> (w539:string[][])
                    }
                    frame 11 {
                      n497 = global read "全局 所有参数.vi" "藻密度"() -> (w540:string[][])
                    }
                  }
                  n498 = Array Size(array=w524) -> (size(s)=w527:i32[])
                  n499 = Index Array(array=w527) -> (element=w526:i32)  [unwired: 1 in]
                  n500 = Greater Than 0?(x=w526) -> (x > 0?=w528:bool)
                  n501 = case shown="真" w528 {
                    tunnel: w526 -> [_ _]
                    tunnel: w524 -> [_ w545]
                    tunnel: [w541 w542] -> w523
                    tunnel: w522 -> [w541 _]
                    frame False {
                    }
                    frame True {
                      # "最新时间戳加1分钟"
                      n502 = Array Size(array=w545) -> (size(s)=w547:i32[])
                      n503 = Index Array(array=w547) -> (element=w546:i32)  [unwired: 1 in]
                      n504 = Decrement(x=w546) -> (x-1=w544:i32)
                      n505 = Index Array(array=w545, index (row)=w544, index (col)=0 ("禁用的索引 (列)")) -> (element=w548:string)
                      n506 = call "日期时间字符串转换分钟数加一.vi"("data[0]"=w548) -> ("日期/时间字符串"=w542:string)  [unwired: 10 in]
                    }
                  }
                }
                n507 = Array To Cluster(array=w518) -> (cluster=w519:T16)
                n508 = global write "全局 时间2.vi" "报警信息索引"(w519) -> ()
              }
            }
          }
          frame #4 {
            # "判定是否存表"
            n509 = global read "全局 数据发送重叠.vi" "掉线指示灯"() -> (w549:bool)
            n510 = case shown="假" w549 {
              frame False {
                # "判定数据不为空才发"
                n511 = global read "全局 数据数组大小.vi" "数据数组大小"() -> (w550:i32)
                n512 = Greater Than 0?(x=w550) -> (x > 0?=w551:bool)
                n513 = case shown="真" w551 {
                  frame False {
                    n514 = global write "全局1.vi" "核查数据上传"(FALSE ("数据上传")) -> ()
                  }
                  frame True {
                    n515 = while {
                      stop <- w554 stop-if-true
                      n516 = Wait (ms)(milliseconds to wait=u32 1000 ("等待时间（毫秒）")) -> ()  [unwired: 1 out]
                      n517 = Get Date/Time In Seconds() -> (seconds since 1Jan1904=w566:timestamp)
                      n518 = Format Date/Time String(time format string (%c)="%Y%m%d%H%M%S%3u" ("时间格式字符串(%c)"), seconds (now)=w566) -> (date/time string=w565:string)  [unwired: 1 in]
                      n519 = global read "全局 数据数组大小.vi" "数据数组大小"() -> (w556:i32)
                      n520 = Search and Replace String(input string=w565, search string="." ("搜索字符串")) -> (result string=w563:string)  [unwired: 6 in, 3 out]
                      n521 = global read "断电保存全局.vi" "PW"() -> (w559:string)
                      n522 = global read "断电保存全局.vi" "MN"() -> (w560:string)
                      n523 = global read "全局 小时数据发送次数.vi" "小时数据发送次数"() -> (w557:i32)
                      n524 = call "数据编码.vi"("table输入"="报警信息" ("新元素/子数组"), "QN"=w563, "MN"=w560, "PW"=w559) -> ("错误常量"=w558:errorcluster, "通讯包字符串"=w562:string)  [unwired: 10 in]
                      n525 = Decrement(x=w556) -> (x-1=w555:i32)
                      n526 = global write "全局1.vi" "发送报文显示"(w562) -> ()
                      n527 = Greater Or Equal?(x=w557, y=w555) -> (x >= y?=w554:bool)
                      n528 = call "通信状态入队列.vi"("错误输入（无错误）"=w558, "枚举"=enum16{"打开连接", "发送数据", "读取数据", "数据处理", "关闭连接"}."发送数据") -> ()  [unwired: 9 in, 1 out]
                    }
                  }
                }
              }
              frame True {
              }
            }
          }
        }
        n529 = global read "断电保存全局.vi" "应用环境"() -> (w505:enum16{"STD", "GB212"})
        n530 = case shown="\"GB212\"" w505 {
          tunnel: ["3093报警信息" ("组合框") w508] -> w504
          frame "STD", Default {
          }
          frame "GB212" {
            n531 = global read "断电保存全局.vi" "仪器参数发送"() -> (w507:bool)
            n532 = case shown="假" w507 {
              tunnel: ["环境参数" ("组合框") "仪器参数" ("组合框")] -> w508
              frame False {
              }
              frame True {
              }
            }
          }
        }
      }
      frame "3093报警信息" {
        # "间隔时间上传"
        # "直接1分钟查询 一次,有数据就按数据上传,没数据为空的不传,在数据发送那边有做处理"
        n533 = flat-sequence {
          tunnel: [w576] -> w571
          tunnel: w571 -> [w580]
          frame #0 {
            n534 = global write "全局 小时数据发送次数.vi" "小时数据发送次数"(0 ("小时数据发送次数")) -> ()
            n535 = global write "全局1.vi" "枚举"(enum16{"返回请求应答", "上传数据", "返回执行结果"}."上传数据" ("枚举")) -> ()
          }
          frame #1 {
            n536 = call "数据表比对.vi"("table输入"="3093报警信息") -> ("待发送数据"=w576:string[][])  [unwired: 7 in, 3 out]
            n537 = global write "全局 所有参数.vi" "CODMn"(w576) -> ()
          }
          frame #2 {
            n538 = Array Size(array=w580) -> (size(s)=w579:i32[])
            n539 = Index Array(array=w579) -> (element=w578:i32)  [unwired: 1 in]
            n540 = global write "全局 数据数组大小.vi" "数据数组大小"(w578) -> ()
          }
          frame #3 {
            n541 = global read "全局 数据发送重叠.vi" "掉线指示灯"() -> (w582:bool)
            n542 = Not(x=w582) -> (.not. x?=w581:bool)
            n543 = case shown="真" w581 {
              frame False {
              }
              frame True {
                # "行数大于零"
                n544 = global read "全局 时间2.vi" "3093报警索引起始时间"() -> (w584:string)
                n545 = global read "全局 所有参数.vi" "CODMn"() -> (w585:string[][])
                n546 = Array Size(array=w585) -> (size(s)=w587:i32[])
                n547 = Index Array(array=w587) -> (element=w586:i32)  [unwired: 1 in]
                n548 = Greater Than 0?(x=w586) -> (x > 0?=w588:bool)
                n549 = case shown="真" w588 {
                  tunnel: w586 -> [_ _]
                  tunnel: w585 -> [_ w594]
                  tunnel: [w589 w590] -> w583
                  tunnel: w584 -> [w589 _]
                  frame False {
                  }
                  frame True {
                    # "最新时间戳加1分钟"
                    n550 = Array Size(array=w594) -> (size(s)=w596:i32[])
                    n551 = Index Array(array=w596) -> (element=w595:i32)  [unwired: 1 in]
                    n552 = Decrement(x=w595) -> (x-1=w593:i32)
                    n553 = Index Array(array=w594, index (row)=w593, index (col)=0 ("禁用的索引 (列)")) -> (element=w591:string)
                    n554 = call "日期时间字符串转换秒数加一.vi"("data[0]"=w591) -> ("日期/时间字符串"=w590:string)  [unwired: 10 in]
                  }
                }
                n555 = global write "全局 时间2.vi" "3093报警索引起始时间"(w583) -> ()
              }
            }
          }
          frame #4 {
            # "判定是否存表"
            n556 = global read "全局 数据发送重叠.vi" "掉线指示灯"() -> (w597:bool)
            n557 = case shown="假" w597 {
              frame False {
                n558 = global read "全局 数据数组大小.vi" "数据数组大小"() -> (w598:i32)
                n559 = Greater Than 0?(x=w598) -> (x > 0?=w599:bool)
                n560 = case shown="真" w599 {
                  frame False {
                  }
                  frame True {
                    n561 = while {
                      stop <- w601 stop-if-true
                      n562 = global read "全局 数据数组大小.vi" "数据数组大小"() -> (w603:i32)
                      n563 = Wait (ms)(milliseconds to wait=u32 1000 ("等待时间（毫秒）")) -> ()  [unwired: 1 out]
                      n564 = global read "全局 小时数据发送次数.vi" "小时数据发送次数"() -> (w602:i32)
                      n565 = Decrement(x=w603) -> (x-1=w604:i32)
                      n566 = Greater Or Equal?(x=w602, y=w604) -> (x >= y?=w601:bool)
                      n567 = Get Date/Time In Seconds() -> (seconds since 1Jan1904=w613:timestamp)
                      n568 = Format Date/Time String(time format string (%c)="%Y%m%d%H%M%S%3u" ("时间格式字符串(%c)"), seconds (now)=w613) -> (date/time string=w612:string)  [unwired: 1 in]
                      n569 = Search and Replace String(input string=w612, search string="." ("搜索字符串")) -> (result string=w610:string)  [unwired: 6 in, 3 out]
                      n570 = global read "断电保存全局.vi" "MN"() -> (w607:string)
                      n571 = global read "断电保存全局.vi" "PW"() -> (w606:string)
                      n572 = call "数据编码.vi"("table输入"="3093报警信息" ("新元素/子数组"), "QN"=w610, "MN"=w607, "PW"=w606) -> ("错误常量"=w605:errorcluster, "通讯包字符串"=w609:string)  [unwired: 10 in]
                      n573 = call "通信状态入队列.vi"("错误输入（无错误）"=w605, "枚举"=enum16{"打开连接", "发送数据", "读取数据", "数据处理", "关闭连接"}."发送数据") -> ()  [unwired: 9 in, 1 out]
                      n574 = global write "全局1.vi" "发送报文显示"(w609) -> ()
                    }
                  }
                }
              }
              frame True {
              }
            }
          }
        }
        n575 = global read "断电保存全局.vi" "仪器参数发送"() -> (w570:bool)
        n576 = case shown="假" w570 {
          tunnel: ["环境参数" ("组合框") "仪器参数" ("组合框")] -> w569
          frame False {
          }
          frame True {
          }
        }
      }
      frame "仪器参数" {
        n577 = flat-sequence {
          frame #0 {
            n578 = global write "全局 小时数据发送次数.vi" "小时数据发送次数"(0 ("小时数据发送次数")) -> ()
            n579 = global write "全局1.vi" "枚举"(enum16{"返回请求应答", "上传数据", "返回执行结果"}."上传数据" ("枚举")) -> ()
          }
          frame #1 {
            n580 = call "获取操作日志 (子VI).vi"("table输入"="仪器参数") -> ()  [unwired: 11 in]
          }
          frame #2 {
            n581 = global read "全局 数据发送重叠.vi" "掉线指示灯"() -> (w621:bool)
            n582 = Not(x=w621) -> (.not. x?=w620:bool)
            n583 = case shown="真" w620 {
              frame False {
              }
              frame True {
                n584 = global read "全局 时间2.vi" "仪器参数索引"() -> (w625:T17)
                n585 = Cluster To Array(cluster=w625) -> (array=w624:string[])
                n586 = for {
                  tunnel: [w629] -> w622 mode=indexing
                  tunnel: w624 -> [w628] mode=indexing
                  i -> [w627]
                  # "行数大于零"
                  n587 = case shown="12" w627 {
                    tunnel: [w633 w634 w635 w636 w637 w638 w639 w640 w641 w642 w643 w644 w645] -> w626
                    frame 0, Default {
                      n588 = global read "全局 所有参数.vi" "氨氮"() -> (w633:string[][])
                    }
                    frame 1 {
                      n589 = global read "全局 所有参数.vi" "总磷"() -> (w634:string[][])
                    }
                    frame 2 {
                      n590 = global read "全局 所有参数.vi" "总氮"() -> (w635:string[][])
                    }
                    frame 3 {
                      n591 = global read "全局 所有参数.vi" "CODMn"() -> (w636:string[][])
                    }
                    frame 4 {
                      n592 = global read "全局 所有参数.vi" "CODCr"() -> (w637:string[][])
                    }
                    frame 5 {
                      n593 = global read "全局 所有参数.vi" "DO"() -> (w638:string[][])
                    }
                    frame 6 {
                      n594 = global read "全局 所有参数.vi" "PH"() -> (w639:string[][])
                    }
                    frame 7 {
                      n595 = global read "全局 所有参数.vi" "电导率"() -> (w640:string[][])
                    }
                    frame 8 {
                      n596 = global read "全局 所有参数.vi" "水温"() -> (w641:string[][])
                    }
                    frame 9 {
                      n597 = global read "全局 所有参数.vi" "浊度"() -> (w642:string[][])
                    }
                    frame 10 {
                      n598 = global read "全局 所有参数.vi" "叶绿素"() -> (w643:string[][])
                    }
                    frame 11 {
                      n599 = global read "全局 所有参数.vi" "藻密度"() -> (w644:string[][])
                    }
                    frame 12 {
                      n600 = global read "全局 所有参数.vi" "ORP"() -> (w645:string[][])
                    }
                  }
                  n601 = Array Size(array=w626) -> (size(s)=w631:i32[])
                  n602 = Index Array(array=w631) -> (element=w630:i32)  [unwired: 1 in]
                  n603 = Greater Than 0?(x=w630) -> (x > 0?=w632:bool)
                  n604 = case shown="真" w632 {
                    tunnel: w630 -> [_ _]
                    tunnel: w626 -> [_ w651]
                    tunnel: [w646 w648] -> w629
                    tunnel: w628 -> [w646 _]
                    frame False {
                    }
                    frame True {
                      # "最新时间戳加1秒"
                      n605 = Array Size(array=w651) -> (size(s)=w653:i32[])
                      n606 = Index Array(array=w653) -> (element=w652:i32)  [unwired: 1 in]
                      n607 = Decrement(x=w652) -> (x-1=w650:i32)
                      n608 = Index Array(array=w651, index (row)=w650, index (col)=0 ("禁用的索引 (列)")) -> (element=w654:string)
                      n609 = call "日期时间字符串转换分钟数加一.vi"("枚举"=enum16{"分钟数加一", "秒数加一", "小时数加一"}."秒数加一", "data[0]"=w654) -> ("日期/时间字符串"=w648:string)  [unwired: 9 in]
                    }
                  }
                }
                n610 = Array To Cluster(array=w622) -> (cluster=w623:T18)
                n611 = global write "全局 时间2.vi" "仪器参数索引"(w623) -> ()
              }
            }
          }
          frame #3 {
            n612 = global read "全局 数据发送重叠.vi" "掉线指示灯"() -> (w656:bool)
            n613 = Not(x=w656) -> (.not. x?=w655:bool)
            n614 = case shown="真" w655 {
              frame False {
              }
              frame True {
                n615 = call "3020仪器参数发送.vi"() -> ()  [unwired: 12 in]
              }
            }
          }
        }
      }
      frame "环境参数", Default {
        n616 = call "核查数据断电保存 (子VI).vi"() -> ()  [unwired: 12 in]
      }
    }
  }
  "错误输出" <- w2
